vi "Record Images.vi"(7 "PPT Path":path, 8 "error in (no error)":errorcluster, 10 "Slide Output path":path, 11 "Slide Information in":T1) -> (0 "error out":errorcluster, 3 "Slide Information out":T1)   [LabVIEW 2015]
uses:
  Slide Info..cluster.ctl
  <vilib>/regexp/Match Regular Expression.xnode
  <vilib>/zip/NI_Unzip.lvlib
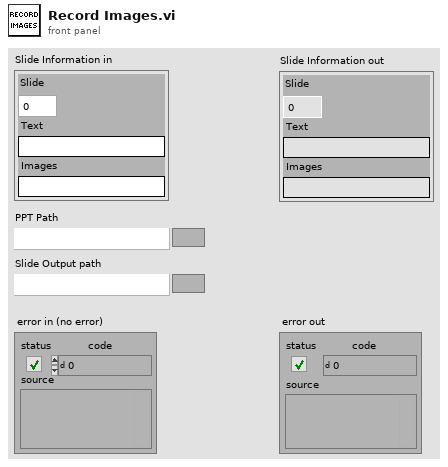
[diagram p1: front panel]
types:
  T1 = typedef "Slide Info..cluster.ctl" = cluster{"Slide":i32, "Text":string, "Images":string}
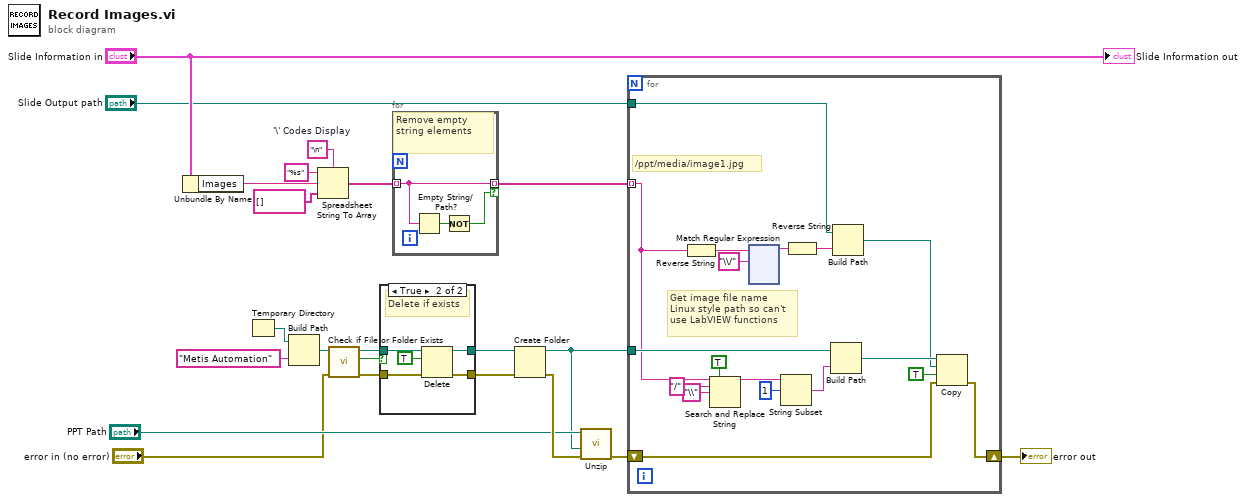
[diagram p0: block diagram]
diagram:
  w19 = "\n"  # '\' Codes Display
  n1 = Unbundle By Name("Slide Information in") -> ("Images"=w21:string)
  n2 = Temporary Directory() -> (w8:path)
  n3 = Build Path(base path=w8, name or relative path="Metis Automation") -> (appended path=w10:path)
  n4 = Spreadsheet String To Array(delimiter (Tab)=w19, format string="%s", spreadsheet string=w21, array type (2D Dbl)=string[] []) -> (array=w17:string[])
  n5 = call <vilib>:"Check if File or Folder Exists.vi"("error in (no error)"="error in (no error)", "path"=w10) -> ("error out"=w13:errorcluster, "file or folder exists?"=w12:bool, "dup path"=w11:path)  [unwired: 7 in]
  n6 = case shown="True" w12 {
    tunnel: w11 -> [w23 w29]
    tunnel: w13 -> [w24 w28]
    tunnel: [w24 w27] -> w15
    tunnel: [w23 w26] -> w14
    frame False {
    }
    frame True {
      # "Delete if exists"
      n7 = Delete(path (use dialog)=w29, entire hierarchy (F)=TRUE, error in=w28) -> (deleted path=w26:path, error out=w27:errorcluster)  [unwired: 2 in, 1 out]
    }
  }
  n8 = for {
    tunnel: w17 -> [w31] mode=indexing
    tunnel: [w31] -> w6 mode=indexing if=w30
    # "Remove empty string elements"
    n9 = Empty String/Path?(string/path=w31) -> (empty?=w32:bool)
    n10 = Not(x=w32) -> (.not. x?=w30:bool)
  }
  n11 = Create Folder(path (use dialog)=w14, error in=w15) -> (created path=w5:path, error out=w16:errorcluster)  [unwired: 1 in, 1 out]
  n12 = call <vilib>:"Unzip.vi"("error in (no error)"=w16, "Target directory (same as Zip file if empty)"=w5, "Zip file"="PPT Path") -> ("error out"=w4:errorcluster)  [unwired: 6 in, 2 out]
  n13 = for {
    tunnel: w6 -> [w44] mode=indexing
    tunnel: w5 -> [w50]
    tunnel: "Slide Output path" -> [w49]
    shift-right: [w33] -> w2
    shift-left: w4 -> [w34]
    # "Get image file name\nLinux style path so can't\nuse LabVIEW functions"
    # "/ppt/media/image1.jpg"
    n14 = Reverse String(1:w44) -> (0:w48:string)
    n15 = Search and Replace String(replace all?=TRUE ("replace all? (F)"), input string=w44, search string="/", replace string="\\" ("replace string (\"\")")) -> (result string=w39:string)  [unwired: 4 in, 3 out]
    n16 = xnode "Match Regular Expression"("input string"=w48, "regular expression"="\\/") -> ("before match"=w46:string)  [unwired: 4 in, 4 out]
    n17 = String Subset(string=w39, offset (0)=1) -> (substring=w38:string)  [unwired: 1 in]
    n18 = Reverse String(1:w46) -> (0:w45:string)
    n19 = Build Path(base path=w50, name or relative path=w38) -> (appended path=w37:path)
    n20 = Build Path(base path=w49, name or relative path=w45) -> (appended path=w36:path)
    n21 = Copy(8:w34, 9:TRUE ("overwrite (F)"), 10:w36, 11:w37) -> (0:w33:errorcluster)  [unwired: 1 in, 2 out]
  }
  "error out" <- w2
  "Slide Information out" <- "Slide Information in"
